vi "2_Regeneration.vi"() -> ()   [LabVIEW 2015]
uses:
  <vilib>/DAQmx/write.llb/DAQmx Write (Analog Wfm 1Chan NSamp).vi
  <vilib>/DAQmx/read.llb/DAQmx Read (Analog DBL 1Chan 1Samp).vi
  <vilib>/DAQmx/create/channels.llb/DAQmx Create Channel (AI-Voltage-Basic).vi
  <vilib>/DAQmx/create/channels.llb/DAQmx Create Channel (AO-Voltage-Basic).vi
  <vilib>/DAQmx/configure/timing.llb/DAQmx Timing (Sample Clock).vi
  <vilib>/DAQmx/miscellaneous.llb/DAQmx Fill In Error Info.vi
  <vilib>/measure/NI_MABase.lvlib
  <resource>/objmgr/daqmx.rc
panel:
  in  "FIFO":bool
  in  "RegenMode":i32(ring)=10158 items=["Allow Regeneration"=10097, "Do Not Allow Regeneration"=10158]
  in  "AI Voltage":tag="myDAQ1/ai0"
  in  "stop":bool
  out "Waveform Chart":dbl(graph)
  in  "AO Voltage":tag
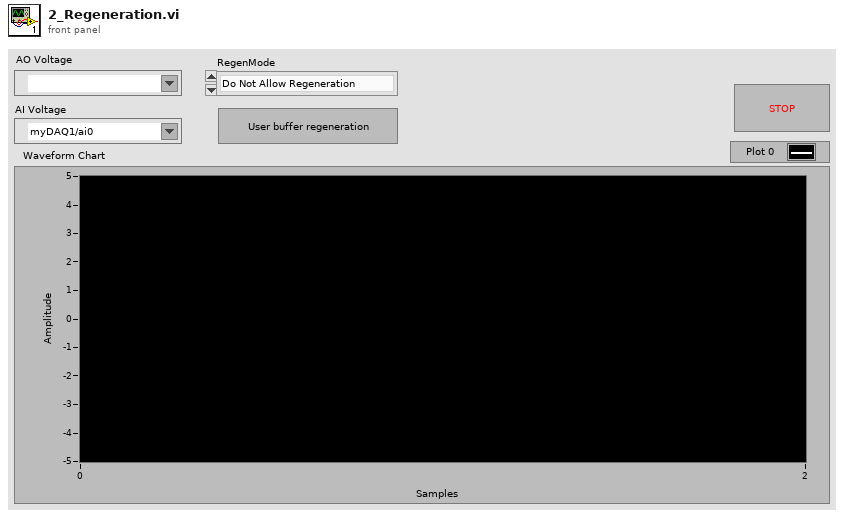
[diagram p1: front panel]
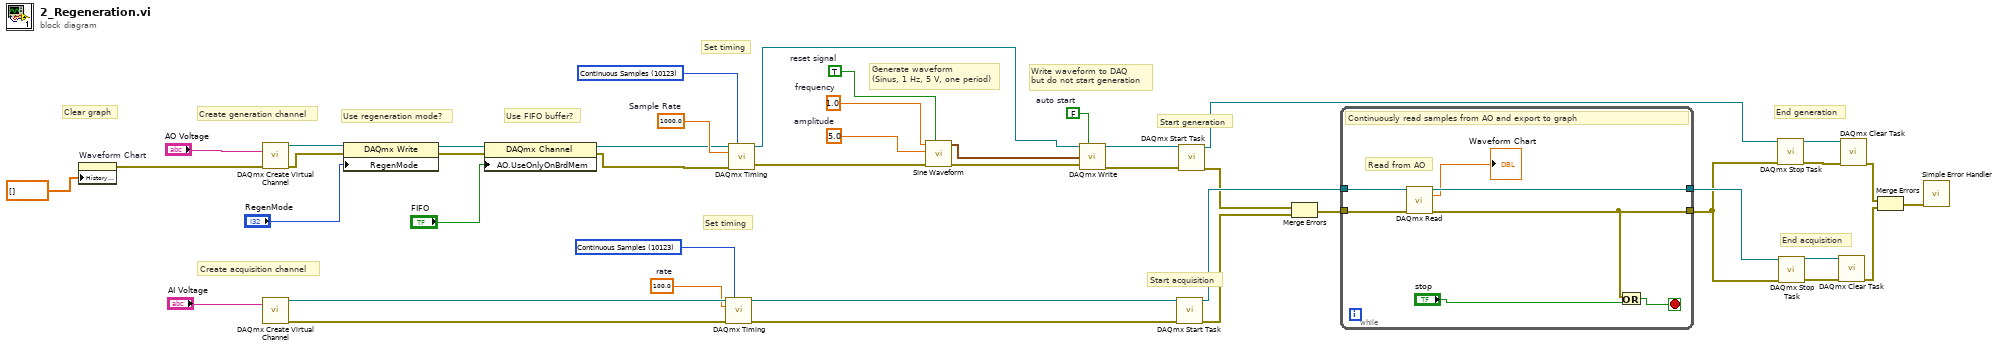
[diagram p0: block diagram]
diagram:
  w12 = 10123 items=["Finite Samples"=10178, "Continuous Samples"=10123, "Hardware Timed Single Point"=12522] ("sample mode")
  w23 = TRUE  # reset signal
  w25 = 5.0  # amplitude
  w26 = 1.0  # frequency
  w41 = 1000.0  # Sample Rate
  w27 = 100.0  # rate
  w39 = FALSE  # auto start
  w40 = 10123 items=["Finite Samples"=10178, "Continuous Samples"=10123, "Hardware Timed Single Point"=12522] ("sample mode")
  # "Clear graph"
  # "Create acquisition channel"
  # "Create generation channel"
  # "Use regeneration mode?"
  # "Use FIFO buffer?"
  # "Set timing"
  # "Set timing"
  # "Write waveform to DAQ\nbut do not start generation"
  # "Generate waveform\n(Sinus, 1 Hz, 5 V, one period)"
  # "End acquisition"
  # "End generation"
  # "Start acquisition"
  # "Start generation"
  n1 = property on="Waveform Chart" class="WFChart (strict)"("History Data"=dbl[] []) -> (error out=w11:errorcluster)  [unwired: 2 in, 1 out]
  n2 = call-poly <vilib>:"DAQmx Create Virtual Channel.vi"("physical channels"="AO Voltage", "error in"=w11) -> ("task out"=w9:refnum<k21>, "error out"=w8:errorcluster)  [unwired: 12 in]
  n3 = call-poly <vilib>:"DAQmx Create Virtual Channel.vi"("physical channels"="AI Voltage") -> ("task out"=w31:refnum<k21>, "error out"=w30:errorcluster)  [unwired: 13 in]
  n4 = property class="DAQmx Write"(reference=w9, error in=w8, "RegenMode"="RegenMode") -> (reference out=w5:refnum<k21>, error out=w4:errorcluster)
  n5 = property class="DAQmx Channel"(reference=w5, error in=w4, "AO.UseOnlyOnBrdMem"="FIFO") -> (reference out=w3:refnum<k21>, error out=w2:errorcluster)
  n6 = call-poly <vilib>:"DAQmx Timing.vi"("task/channels in"=w31, "sample mode"=w12, "rate"=w27, "error in"=w30) -> ("task out"=w29:refnum<k21>, "error out"=w28:errorcluster)  [unwired: 10 in]
  n7 = call-poly <vilib>:"DAQmx Timing.vi"("task/channels in"=w3, "sample mode"=w40, "rate"=w41, "error in"=w2) -> ("task out"=w1:refnum<k21>, "error out"=w22:errorcluster)  [unwired: 10 in]
  n8 = call <vilib>:"Sine Waveform.vi"("reset signal"=w23, "error in (no error)"=w22, "amplitude"=w25, "frequency"=w26) -> ("error out"=w21:errorcluster, "signal out"=w24:waveform(dbl))  [unwired: 6 in]
  n9 = call-poly <vilib>:"DAQmx Write.vi"("task/channels in"=w1, "auto start"=w39, "data"=w24, "error in"=w21) -> ("task out"=w44:refnum<k21>, "error out"=w32:errorcluster)  [unwired: 9 in, 1 out]
  n10 = call <vilib>:"DAQmx Start Task.vi"("task/channels in"=w29, "error in"=w28) -> ("task out"=w36:refnum<k21>, "error out"=w19:errorcluster)  [unwired: 12 in]
  n11 = call <vilib>:"DAQmx Start Task.vi"("task/channels in"=w44, "error in"=w32) -> ("task out"=w6:refnum<k21>, "error out"=w20:errorcluster)  [unwired: 12 in]
  n12 = Merge Errors(w20, w19) -> (w13:errorcluster)
  n13 = while {
    tunnel: w36 -> [w51]
    tunnel: [w50] -> w35
    tunnel: w13 -> [w46]
    tunnel: [w45] -> w18
    stop <- w47 stop-if-true
    # "Read from AO"
    # "Continuously read samples from AO and export to graph"
    n14 = call-poly <vilib>:"DAQmx Read.vi"("task/channels in"=w51, "error in"=w46) -> ("task out"=w50:refnum<k21>, "data"=→"Waveform Chart":dbl, "error out"=w45:errorcluster)  [unwired: 11 in]
    n15 = Or(x=w45, y="stop") -> (x .or. y?=w47:bool)
  }
  n16 = call <vilib>:"DAQmx Stop Task.vi"("task/channels in"=w6, "error in"=w18) -> ("task out"=w43:refnum<k21>, "error out"=w42:errorcluster)  [unwired: 12 in]
  n17 = call <vilib>:"DAQmx Stop Task.vi"("task/channels in"=w35, "error in"=w18) -> ("task out"=w33:refnum<k21>, "error out"=w34:errorcluster)  [unwired: 12 in]
  n18 = call <vilib>:"DAQmx Clear Task.vi"("task in"=w33, "error in"=w34) -> ("error out"=w16:errorcluster)  [unwired: 13 in]
  n19 = call <vilib>:"DAQmx Clear Task.vi"("task in"=w43, "error in"=w42) -> ("error out"=w17:errorcluster)  [unwired: 13 in]
  n20 = Merge Errors(w17, w16) -> (w15:errorcluster)
  n21 = call <vilib>:"Simple Error Handler.vi"("error in (no error)"=w15) -> ()  [unwired: 4 in, 5 out]
